vi "action.vi"(0 "HGF_SVVisitor_runMon in":refnum<class "HGF_SVMonitorVisitor_getReg.lvclass">, 2 "HGF_Visitable":refnum<class "HGF_Visitable.lvclass">, 5 "error in (no error)":errorcluster) -> (14 "HGF_SVVisitor_runMon out":refnum<class "HGF_SVMonitorVisitor_getReg.lvclass">, 16 "dup HGF_Visitable":refnum<class "HGF_Visitable.lvclass">, 19 "error out":errorcluster)   [LabVIEW 2012, in "HGF_SV.lvlib" / "HGF_SVMonitorVisitor_getReg.lvclass"]
doc: "This is a dynamic dispatch VI that is called from Visitor.visit(). It will call member VIs of Visitable to perform the requested action which means: calling public methods of Visitable child class.\n\n<B>Hint:</B> This method is abstract and need to be implemented by child classes."
uses:
  HGF_SVMonitorVisitor_getReg.lvclass
  HGF_BaseClasses/HGF_Visitable/HGF_Visitable.lvclass
  HGF_BaseClasses/HGF_Visitor/HGF_Visitor.lvclass
  HGF_Monitor/HGF_Monitor.lvclass
  HGF_SVMonitorVisitor_getReg.lvclass/HGF_SVMonitorVisitor_getReg.ctl
  HGF_SVMonitorVisitor/HGF_SVMonitorVisitor.lvclass
  HGF_BaseClasses/HGF_TriggeredEvent/HGF_TriggeredEvent.lvclass
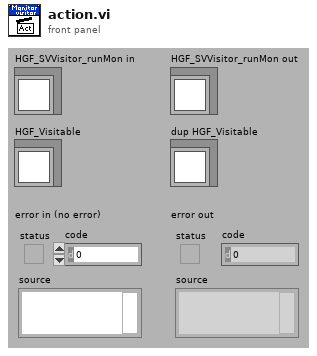
[diagram p1: front panel]
types:
  T1 = cluster{"URL":string, "registered Visitors":cluster{"HGF_NetworkVisitor":refnum<class "HGF_NetworkVisitor.lvclass">, "HGF_TriggeredEvent":refnum<class "HGF_TriggeredEvent.lvclass">}[]}[]
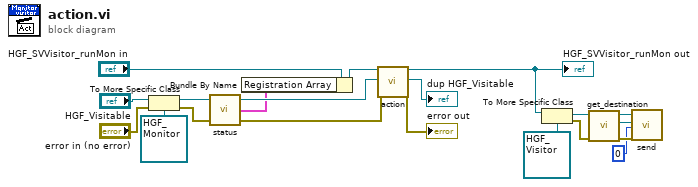
[diagram p0: block diagram]
diagram:
  n1 = To More Specific Class(target class=refnum<class "HGF_Monitor.lvclass"> refnum ("HGF_SV.lvlib:HGF_Monitor.lvclass"), reference="HGF_Visitable", error in="error in (no error)") -> (specific class reference=w6:refnum<class "HGF_Monitor.lvclass">, error out=w5:errorcluster)
  n2 = call-dynamic "status.vi"("error in (no error)"=w5, "HGF_Monitor in"=w6) -> ("error out"=w3:errorcluster, "Array"=w2:T1, "HGF_Monitor out"=w4:refnum<class "HGF_Monitor.lvclass">)  [unwired: 1 in]
  n3 = Bundle By Name(cluster="HGF_SVVisitor_runMon in", "Registration Array"=w2) -> (w15:refnum<class "HGF_SVMonitorVisitor_getReg.lvclass">)
  n4 = call-parent "action.vi"("HGF_SVVisitor_runMon in"=w15, "HGF_Visitable"=w4, "error in (no error)"=w3) -> ("HGF_SVVisitor_runMon out"=w14:refnum<class "HGF_SVMonitorVisitor_getReg.lvclass">, "dup HGF_Visitable"=→"dup HGF_Visitable":refnum<class "HGF_Visitable.lvclass">, "error out"=→"error out":errorcluster)  [unwired: 14 in]
  "HGF_SVVisitor_runMon out" <- w14
  n5 = To More Specific Class(target class=refnum<class "HGF_Visitor.lvclass"> refnum ("HGF_BaseClasses.lvlib:HGF_Visitor.lvclass"), reference=w14) -> (specific class reference=w12:refnum<class "HGF_Visitor.lvclass">, error out=w11:errorcluster)  [unwired: 1 in]
  n6 = call "get_destination.vi"("error in (no error)"=w11, "HGF_Visitor"=w12) -> ("error out"=w8:errorcluster, "destination"=w9:refnum<class "HGF_TriggeredEvent.lvclass">, "dup HGF_Visitor"=w10:refnum<class "HGF_Visitor.lvclass">)  [unwired: 7 in]
  n7 = call-dynamic "send.vi"("HGF_Event"=w9, "Object"=w10, "timeout in ms (-1)"=0, "error in (no error)"=w8) -> ()  [unwired: 13 in, 3 out]
